vi "obtain_latest_instance.vi"(7 "quick, but maybe outdated?":bool=TRUE, 8 "error in (no error)":errorcluster) -> (0 "error out":errorcluster, 3 "GenericScanMode out":refnum<class "GenericImagingMode.lvclass">)   [LabVIEW 2010, in "GenericImagingMode.lvclass"]
uses:
  GenericImagingMode.lvclass
  class_data.vi
  common/classes/ErrorController/ErrorController/class_data.vi
  common/classes/ErrorController/ErrorController/ErrorController.lvclass
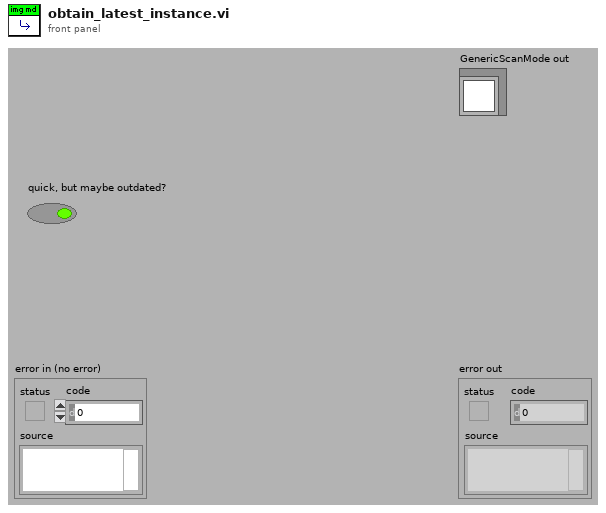
[diagram p1: front panel]
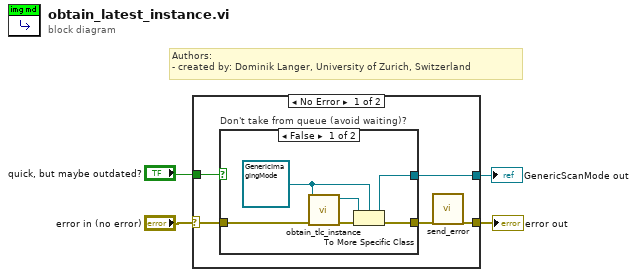
[diagram p0: block diagram]
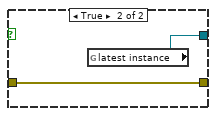
[diagram p2: hidden frame]
diagram:
  # "Authors: \n- created by: Dominik Langer, University of Zurich, Switzerland"
  n1 = case shown="No Error" "error in (no error)" {
    selector: "error in (no error)" -> [w9 w18]
    tunnel: [w5 w18] -> w3
    tunnel: [w8 _] -> w2
    tunnel: "quick, but maybe outdated?" -> [w7 _]
    frame No Error {
      n2 = case "Don't take from queue (avoid waiting)?" shown="False" w7 {
        tunnel: w9 -> [w11 w17]
        tunnel: [w14 w17] -> w6
        tunnel: [w12 w16] -> w8
        frame False {
          w10 = refnum<class "GenericImagingMode.lvclass"> refnum ("GenericScanMode.lvclass")
          n3 = call-dynamic "obtain_tlc_instance.vi"("error in (no error)"=w11, "GenericToplevelComponent in"=w10) -> ("error out"=w15:errorcluster, "GenericToplevelComponent out"=w13:refnum<class "GenericToplevelComponent.lvclass">)  [unwired: 8 in]
          n4 = To More Specific Class(target class=w10, reference=w13, error in=w15) -> (specific class reference=w12:refnum<class "GenericImagingMode.lvclass">, error out=w14:errorcluster)
        }
        frame True {
          n5 = global read "class_data.vi" "latest instance"() -> (w16:refnum<class "GenericImagingMode.lvclass">)
        }
      }
      n6 = call "send_error.vi"("error in (no error)"=w6) -> ("error out"=w5:errorcluster)  [unwired: 10 in]
    }
    frame Error {
    }
  }
  "error out" <- w3
  "GenericScanMode out" <- w2
